vi "vectornav test.vi"() -> ()   [LabVIEW 2009]
uses:
  <vilib>/Instr/_visa.llb/VISA Configure Serial Port (Instr).vi
panel:
  in  "stop":bool
  in  "manual data":string
  in  "live data?":bool
  in  "VISA resource name":refnum<visa-resource-name>="COM4"
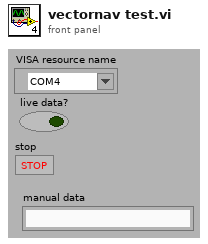
[diagram p1: front panel]
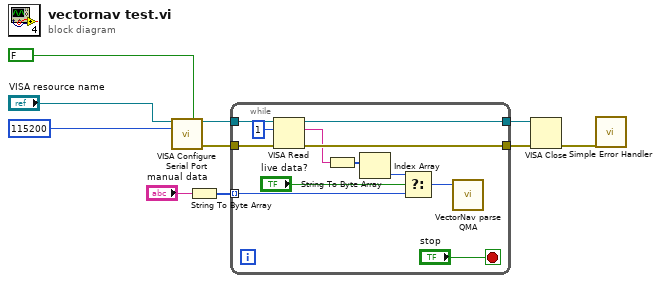
[diagram p0: block diagram]
diagram:
  n1 = call-poly "VISA Configure Serial Port"("VISA resource name"="VISA resource name", "Enable Termination\nChar (T)"=FALSE ("Enable Termination\nChar (T)"), "baud rate (9600)"=u32 115200) -> ("VISA resource name out"=w7:refnum<visa-resource-name>, "error out"=w6:errorcluster)  [unwired: 6 in, 5 out]
  n2 = String To Byte Array(string="manual data") -> (unsigned byte array=w1:u8[])
  n3 = while {
    tunnel: w7 -> [w22]
    tunnel: w6 -> [w20]
    tunnel: [w18] -> w3
    tunnel: [w17] -> w4
    tunnel: w1 -> [w14] mode=indexing
    stop <- "stop" stop-if-true
    n4 = VISA Read(VISA resource name=w22, byte count=u32 1, error in (no error)=w20) -> (VISA resource name out=w18:refnum<visa-resource-name>, read buffer=w15:string, error out=w17:errorcluster)  [unwired: 1 out]
    n5 = String To Byte Array(string=w15) -> (unsigned byte array=w13:u8[])
    n6 = Index Array(array=w13) -> (element=w12:u8)  [unwired: 1 in]
    n7 = Select(t=w12, s="live data?", f=w14) -> (s? t:f=w11:u8)
    n8 = call "VectorNav parse QMA.vi"("input data"=w11) -> ()  [unwired: 11 in]
  }
  n9 = VISA Close(VISA resource name=w3, error in (no error)=w4) -> (error out=w5:errorcluster)
  n10 = call <vilib>:"Simple Error Handler.vi"("error in (no error)"=w5) -> ()  [unwired: 1 in, 8 out]
